vi "Iterate Audio.vi"(9 "Chunk size":i32=4096, 11 "Msg":sgl[](array[numeric])) -> (1 "Finished":bool, 3 "Subarray":sgl[](array[numeric]))   [LabVIEW 2015]
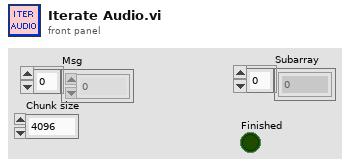
[diagram p1: front panel]
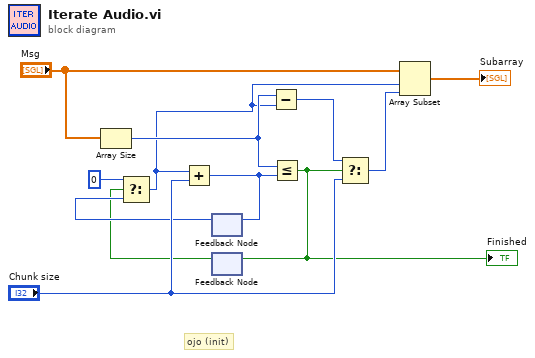
[diagram p0: block diagram]
diagram:
  # "ojo (init)"
  n1 = Array Size(array="Msg") -> (size(s)=w8:i32)
  n2 = feedback #1() -> (w5:i32)  [unwired: 1 in]
  n3 = feedback #2() -> (w4:bool)  [unwired: 1 in]
  n4 = Select(t=0, s=w4, f=w5) -> (s? t:f=w2:i32)
  n5 = Add(x=w2, y="Chunk size") -> (x+y=w12:i32)
  n6 = feedback-in #1(w12) -> ()
  n7 = Subtract(x=w8, y=w2) -> (x-y=w11:i32)
  n8 = Less Or Equal?(x=w8, y=w12) -> (x <= y?=w6:bool)
  "Finished" <- w6
  n9 = feedback-in #2(w6) -> ()
  n10 = Select(t=w11, s=w6, f="Chunk size") -> (s? t:f=w9:i32)
  n11 = Array Subset(array="Msg", index=w2, length=w9) -> (→"Subarray":sgl[])
